vi "SetInstrumentFromMarker.vi"(8 "error in (no error)":errorcluster, 11 "Keysight44xx in":refnum<class "Keysight44xx.lvclass">) -> (0 "error out":errorcluster, 3 "Keysight44xx out":refnum<class "Keysight44xx.lvclass">)   [LabVIEW 2018, in "SpecAnPlugins.lvlib" / "Keysight44xx.lvclass"]
doc: "This VI makes the Active Marker frequency to be the start frequency, the stop frequency, or the center frequency. It can also make the active marker amplitude to be the reference level. This affects either the Frequency Start, Frequency Stop, or the Reference Level property. \n\nNotes:\n\n(1) This VI INVALIDATES the Frequency Start and Frequency Stop property values or INVALIDATES Reference Level property.\n\n(2) This VI will return error Marker Not Enabled if the active marker is not enabled."
uses:
  Keysight44xx.lvclass
  C:/Users/ico/Documents/Projects/NistPluggableModules/SpecAn/SpecAnPlugins/SpecAnBaseClass/SpecAnBase.lvclass
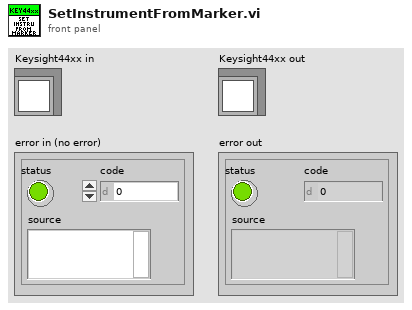
[diagram p1: front panel]
types:
  T1 = typedef "SpecAnPlugins.lvlib/SpecAnBase.lvclass/Acquisition.ctl" = cluster{"Handle":string, "Connected":bool, "Enabled":bool, "SweepModeContinuous":bool, "NumberOfSweeps":i32, "DetectorTypeAuto":bool, "DetectorType":i32, "VerticalScale":i32, "MaximumTime(seconds)":dbl}
  T2 = typedef "SpecAnPlugins.lvlib/SpecAnBase.lvclass/Markers.ctl" = cluster{"MarkerEnabled":bool, "MarkerThreshold":dbl, "PeakExcursion":dbl, "SignalTrackEnabled":bool, "MarkerPosition":dbl, "Instrument Setting (Frequency Center)":i32, "Marker search (Minimum)":i32, "ActiveMarker":string, "MarkerFrequencyCounter":bool, "FrequencyCounterResolution":dbl}
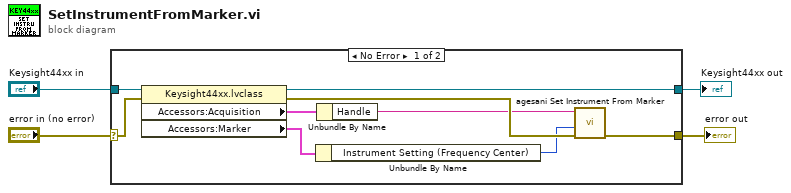
[diagram p0: block diagram]
diagram:
  n1 = case shown="No Error" "error in (no error)" {
    selector: "error in (no error)" -> [w12 w14]
    tunnel: "Keysight44xx in" -> [w13 w15]
    tunnel: [w11 w15] -> w2
    tunnel: [w5 w14] -> w1
    frame No Error {
      n2 = property class="Keysight44xx.lvclass"(reference=w13, error in=w12) -> (reference out=w11:refnum<class "Keysight44xx.lvclass">, error out=w8:errorcluster, "Accessors:Acquisition"=w10:T1, "Accessors:Marker"=w9:T2)
      n3 = Unbundle By Name(w9) -> ("Instrument Setting (Frequency Center)"=w6:i32)
      n4 = Unbundle By Name(w10) -> ("Handle"=w7:string)
      n5 = call <instrlib>:"agesani Set Instrument From Marker.vi"("error in (no error)"=w8, "instrument setting (Frequency Center)"=w6, "instrument handle"=w7) -> ("error out"=w5:errorcluster)  [unwired: 7 in, 1 out]
    }
    frame Error {
    }
  }
  "error out" <- w1
  "Keysight44xx out" <- w2
